vi "Simulation Full Step.vi"(8 "Error In":errorcluster, 10 "iRobot Play Button (false)":bool, 11 "simulator":T1={"configuration"={"maxTime"=5.0, "enableVisualization"=TRUE, "statechart"=path "iRobot Navigation State Machine.vi", "environment"=path "iRobot Navigation State Machine.vi", "record"=path "Simulation Record.xml", "autograde?"=TRUE, "interactive?"=FALSE, "feedback mode"=enum."debug navigation"}, "Bump Sensors"=[], "Distance Sensors"=[], "Accelerometer"=refnum, "Wall Sensor"=refnum, "Statechart\ndisplay"=refnum, "Body"=refnum, "Left Motor"=refnum, "Right Motor"=refnum, "first step?"=FALSE}) -> (0 "Error Out":errorcluster, 1 "continue to next step?":bool, 2 "simulated time (s)":sgl format="%7.3g", 3 "simulator":T1={"configuration"={"maxTime"=5.0, "enableVisualization"=TRUE, "statechart"=path "iRobot Navigation State Machine.vi", "environment"=path "iRobot Navigation State Machine.vi", "record"=path "Simulation Record.xml", "autograde?"=TRUE, "interactive?"=FALSE, "feedback mode"=enum."debug navigation"}, "Bump Sensors"=[], "Distance Sensors"=[], "Accelerometer"=refnum, "Wall Sensor"=refnum, "Statechart\ndisplay"=refnum, "Body"=refnum, "Left Motor"=refnum, "Right Motor"=refnum, "first step?"=FALSE}, 4 "iRobot Sensor Display":T4 {"Right Wheel (mm/s)" scale=-500.0..500.0; "Left Wheel (mm/s)" scale=-500.0..500.0})   [LabVIEW 2013]
uses:
  shared/iRobot Sensor Display.ctl
  Simulator.ctl
  <instrlib>/DC Motor Controller/HAIOL/DC Motor Controller.lvclass
  CyberSim interface/Simulation Configuration.ctl
  autograder/feedbackMode.ctl
  Simulation Call Statechart Operation.ctl
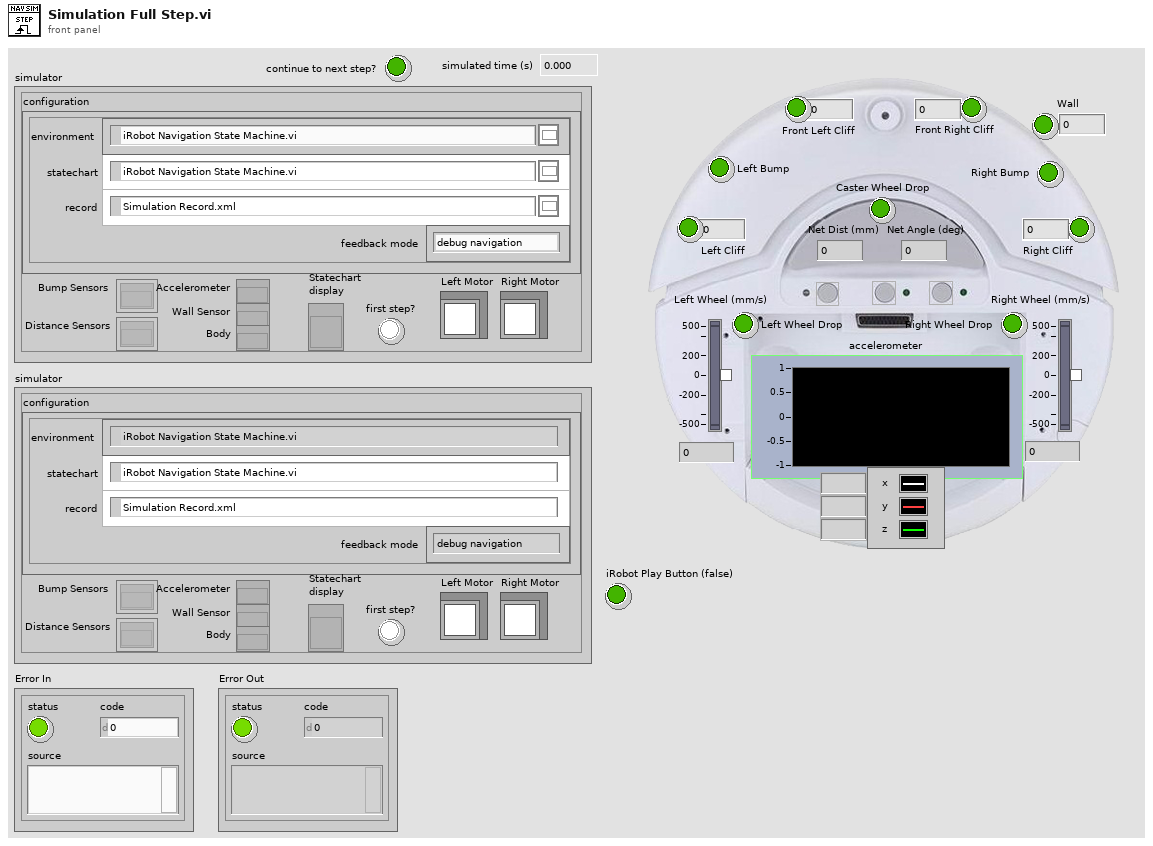
[diagram p1: front panel]
types:
  T1 = typedef "Simulator.ctl" = cluster{"configuration":T2, "Bump Sensors":refnum<k20>[], "Distance Sensors":refnum<k20>[], "Accelerometer":refnum<k20>, "Wall Sensor":refnum<k20>, "Statechart\ndisplay":refnum<vi>, "Body":refnum<k20>, "Left Motor":refnum<class "DC Motor Controller.lvclass">, "Right Motor":refnum<class "DC Motor Controller.lvclass">, "first step?":bool}
  T2 = typedef "Simulation Configuration.ctl" = cluster{"maxTime":sgl, "enableVisualization":bool, "statechart":path, "environment":path, "record":path, "autograde?":bool, "interactive?":bool, "feedback mode":T3}
  T3 = typedef "feedbackMode.ctl" = enum32{"debug navigation", "debug hill climb", "autograde navigation", "autograde hill climb"}
  T4 = typedef "iRobot Sensor Display.ctl" = cluster{"Caster Wheel Drop":bool, "Left Wheel Drop":bool, "Right Wheel Drop":bool, "Left Bump":bool, "Right Bump":bool, "Left Cliff":bool, "Front Left Cliff":bool, "Front Right Cliff":bool, "Right Cliff":bool, "Wall":bool, "Net Dist (mm)":i32, "Net Angle (deg)":i32, "Wall":u16, "Left Cliff":u16, "Front Left Cliff":u16, "Front Right Cliff":u16, "Right Cliff":u16, "Left Wheel (mm/s)":i16, "Right Wheel (mm/s)":i16, "accelerometer":T5}
  T5 = typedef "Accelerometer.ctl" = cluster{"x axis (g)":dbl, "y axis (g)":dbl, "z axis (g)":dbl}
  T6 = typedef "Simulation Call Statechart Operation.ctl" = enum16{"Initialize", "Call Statechart", "Finalize"}
  T7 = typedef "Sensors.ctl" = cluster{"net distance (mm)":i32, "net angle (deg)":i32, "accelerometer":T5, "iRobot Sensors":T8, "Is Simulator?":bool}
  T8 = typedef "Sensor Group 6.ctl" = cluster{"Bumps + Wheel Drops":T9, "Wall":bool, "Cliff Left":bool, "Cliff Front Left":bool, "Cliff Front Right":bool, "Cliff Right":bool, "Wall Signal":u16, "Cliff Left Signal":u16, "Cliff Front Left Signal":u16, "Cliff Front Right Signal":u16, "Cliff Right Signal":u16, "Buttons":T10, "Virtual Wall":bool, "# Stream Packets":u8, "Requested Velocity (mm/s)":i16, "Requested Radius (mm)":i16, "Requested Right Wheel Velocity (mm/s)":i16, "Requested Left Wheel Velocity (mm/s)":i16, "Distance (mm)":i32, "Angle (deg)":i32, "Song Playing":bool, "Song Number":u8, "Charging State":T11, "Voltage (mV)":u16, "Current (mA)":i16, "Battery Temperature (deg C)":i8, "Battery Charge (mAh)":u16, "Battery Capacity (mAh)":u16, "Charging Sources":T12, "OI Mode":T13, "Digital Inputs":T14, "Drivers & Wheel Overcurrent":T15, "Analog Signal":u16, "Infrared":u8}
  T9 = typedef "Bumps + Wheel Drops.ctl" = cluster{"Wheeldrop Caster":bool, "Wheeldrop Left":bool, "Wheeldrop Right":bool, "Bump Left":bool, "Bump Right":bool}
  T10 = typedef "Buttons.ctl" = cluster{"Advance":bool, "Play":bool}
  T11 = typedef "Charging State.ctl" = enum16{"Not Charging", "Reconditioning Charging", "Full Charging", "Trickle Charging", "Waiting", "Charging Fault Condition"}
  T12 = typedef "Charging Sources Available.ctl" = cluster{"Internal Charger":bool, "Home Base":bool}
  T13 = typedef "OI Mode.ctl" = enum16{"Off", "Passive", "Safe", "Full"}
  T14 = typedef "Cargo Bay Digital Inputs.ctl" = cluster{"Digital Input 0":bool, "Digital Input 1":bool, "Digital Input 2":bool, "Digital Input 3":bool, "Device Detect":bool}
  T15 = typedef "Low-Side Driver + Wheel Overcurrent.ctl" = cluster{"Low-Side Driver 0":bool, "Low-Side Driver 1":bool, "Low-Side Driver 2":bool, "Left Wheel":bool, "Right Wheel":bool}
  T16 = typedef "Simulation Trace Element.ctl" = cluster{"sensors":T7, "position":T17, "orientation":T18, "Simulation Time (s)":sgl}
  T17 = typedef "Simulated iRobot Position.ctl" = cluster{"x (m)":sgl, "y (m)":sgl, "z (m)":sgl}
  T18 = typedef "Simulated iRobot Orientation.ctl" = cluster{"roll (deg)":sgl, "pitch (deg)":sgl, "yaw (deg)":sgl}
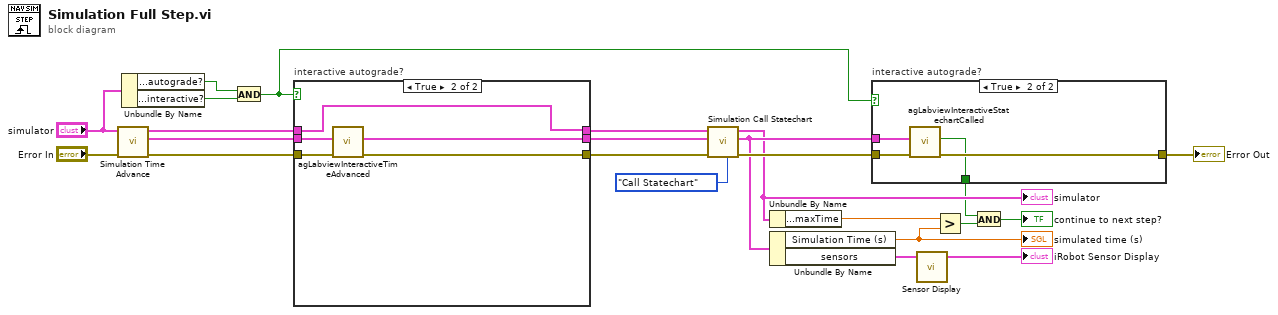
[diagram p0: block diagram]
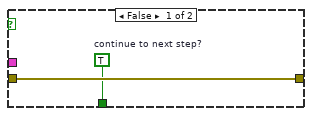
[diagram p2: hidden frame]
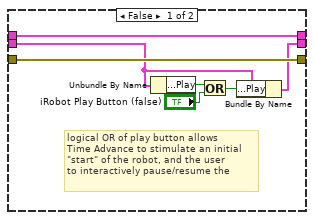
[diagram p3: hidden frame]
diagram:
  n1 = call "Simulation Time Advance.vi"("error in (no error)"="Error In", "simulator"="simulator") -> ("error out"=w12:errorcluster, "sensors"=w13:T7, "simulator"=w14:T1)  [unwired: 7 in]
  n2 = Unbundle By Name("simulator") -> ("configuration.autograde?"=w16:bool, "configuration.interactive?"=w15:bool)
  n3 = And(x=w16, y=w15) -> (x .and. y?=w8:bool)
  n4 = case "interactive autograde?" shown="True" w8 {
    tunnel: w14 -> [w27 w33]
    tunnel: w13 -> [w25 w34]
    tunnel: w12 -> [w26 w35]
    tunnel: [w27 w33] -> w11
    tunnel: [w24 w32] -> w10
    tunnel: [w26 w31] -> w9
    frame False {
      # "logical OR of play button allows\nTime Advance to stimulate an initial\n\"start\" of the robot, and the user\nto interactively pause/resume the"
      n5 = Unbundle By Name(w25) -> ("iRobot Sensors.Buttons.Play"=w28:bool)
      n6 = Or(x=w28, y="iRobot Play Button (false)") -> (x .or. y?=w30:bool)
      n7 = Bundle By Name(cluster=w25, "iRobot Sensors.Buttons.Play"=w30) -> (w24:T7)
    }
    frame True {
      n8 = call "agLabviewInteractiveTimeAdvanced.vi"("Error In"=w35, "sensors"=w34) -> ("Error Out"=w31:errorcluster, "sensors"=w32:T7)  [unwired: 8 in]
    }
  }
  n9 = call "Simulation Call Statechart.vi"("operation"=Simulation_Call_Statechart_Operation."Call Statechart", "error in"=w9, "sensors"=w10, "simulator"=w11) -> ("error out"=w7:errorcluster, "trace element"=w6:T16, "simulator"=w4:T1)  [unwired: 5 in]
  "simulator" <- w4
  n10 = Unbundle By Name(w4) -> ("configuration.maxTime"=w22:sgl)
  n11 = Unbundle By Name(w6) -> ("Simulation Time (s)"=w20:sgl, "sensors"=w19:T7)
  "simulated time (s)" <- w20
  n12 = case "interactive autograde?" shown="True" w8 {
    tunnel: w7 -> [w37 w41]
    tunnel: w6 -> [_ w40]
    tunnel: [w37 w39] -> w5
    tunnel: [w36 w38] -> w2
    frame False {
      w36 = TRUE  # continue to next step?
    }
    frame True {
      n13 = call "agLabviewInteractiveStatechartCalled.vi"("Error In"=w41, "Trace Element"=w40) -> ("Error Out"=w39:errorcluster, "continue to next step?"=w38:bool)  [unwired: 8 in]
    }
  }
  "Error Out" <- w5
  n14 = call "Sensor Display.vi"("sensors"=w19) -> ("irobot sensor display"=→"iRobot Sensor Display":T4)  [unwired: 4 in]
  n15 = Greater?(x=w22, y=w20) -> (0:w3:bool)
  n16 = And(x=w2, y=w3) -> (x .and. y?=→"continue to next step?":bool)
